vi "Configure Save File.vi"(0 "subVI":refnum<vi>, 2 "VI":refnum<vi>, 3 "ParentVI":refnum<vi>) -> (1 "Data Valid":bool)   [LabVIEW 2017]
doc: "Writes data to a LabVIEW measurement data file."
uses:
  <vilib>/express/express shared/ExFile.llb/ex_FileGlobals.vi
panel:
  in  "always hostless warning":string="The present target will not have a host connected.  When run, this VI will return an error."
  in  "maybe hostless warning":string="The present target may not always have a host connected.  When running hostless, this VI will return an error."
  in  "delimiter":string
  in  "x_columns":enum32{"none", "one", "multiple"}(radio)
  in  "overwrite_mode":T1(radio)
  in  "column headings":enum32{"one per segment", "once", "none"}(radio)
  in  "storage_format":enum32{"lvm", "tdm"}(radio)
  in  "delimiter enum":enum32{"tab", "comma"}(radio)
  in  "File path":path
  in  "Ask each iteration":bool
  in  "Ask only once":bool
  in  "Help":bool
  in  "Ok":bool
  in  "Cancel":bool
  in  "overwrite_mode_multi":i32
  in  "fixed_width":bool=TRUE
  in  "Width":i32=2 min=1 max=9
  in  "Samples":i32=1 min=1
  in  "Segments":i32=1 min=1
  in  "new_file_samples":bool
  in  "new_file_iter":bool
  in  "Time":i32 min=0 max=86399 format="%<%I:%M %p\n%m/%d/%y>T"
  in  "new_file_daily":bool
  in  "max_elapsed_seconds":i32 min=0 max=999
  in  "new_file_elaps_time":bool
  in  "KB":i32=100
  in  "new_file_size":bool=TRUE
  in  "Settings":bool
  in  "Save to series of files (multiple files)":bool
  in  "Save to one file":bool=TRUE
  in  "File Description":string
  in  "Ask user to choose file":bool
  in  "multi_file":bool
  in  "time_format_string":string="%Y-%m-%d"
  in  "new_file_mode":u16(ring)=2 items=["Date & Time", "Serial No.", "Both"]
  in  "File name":path=path "test.lvm"
  # "File Format"
  # "File Name"
  # "Action"
  # "Segment Headers"
  # "X Value Columns"
  # "If a file already exists"
  # "Delimiter"
  # "File Description"
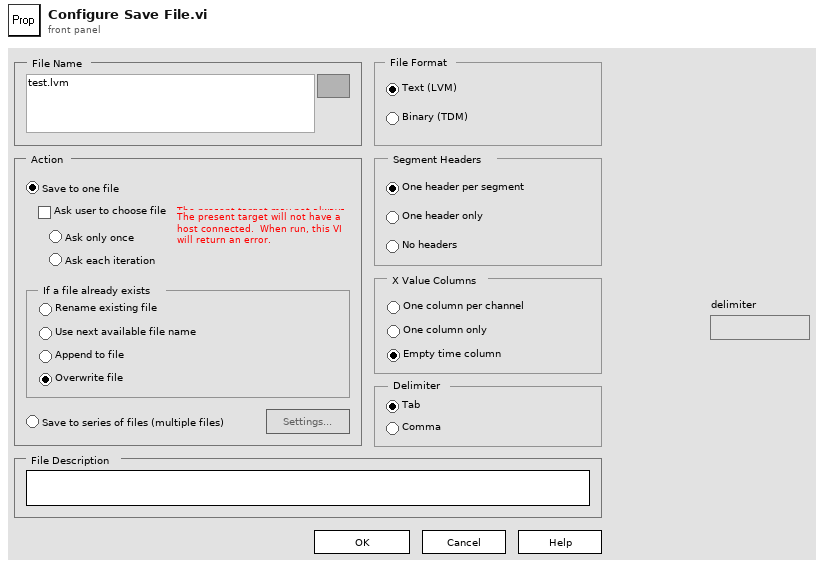
[diagram p1: front panel]
types:
  T1 = enum32{"overwrite", "overwrite & backup", "append", "next avail"}
  T2 = cluster{"Ctl Type":u16, "LV Express VI Ctl Label":string, "Wizard Ctl Label":string}[]
  T3 = typedef "propPageData.ctl" = cluster{"InstanceCtlRefs":refnum<vi>[], "ConfigDlgCtlRefs":refnum<vi>[], "Control Data":cluster{"Ctl Type":u16, "Instance Ctl Label":string, "Config Dialog Ctl Label":string}[], "viref Instance":refnum<vi>, "Types":i32[], "Config DialogVI":refnum<vi>}
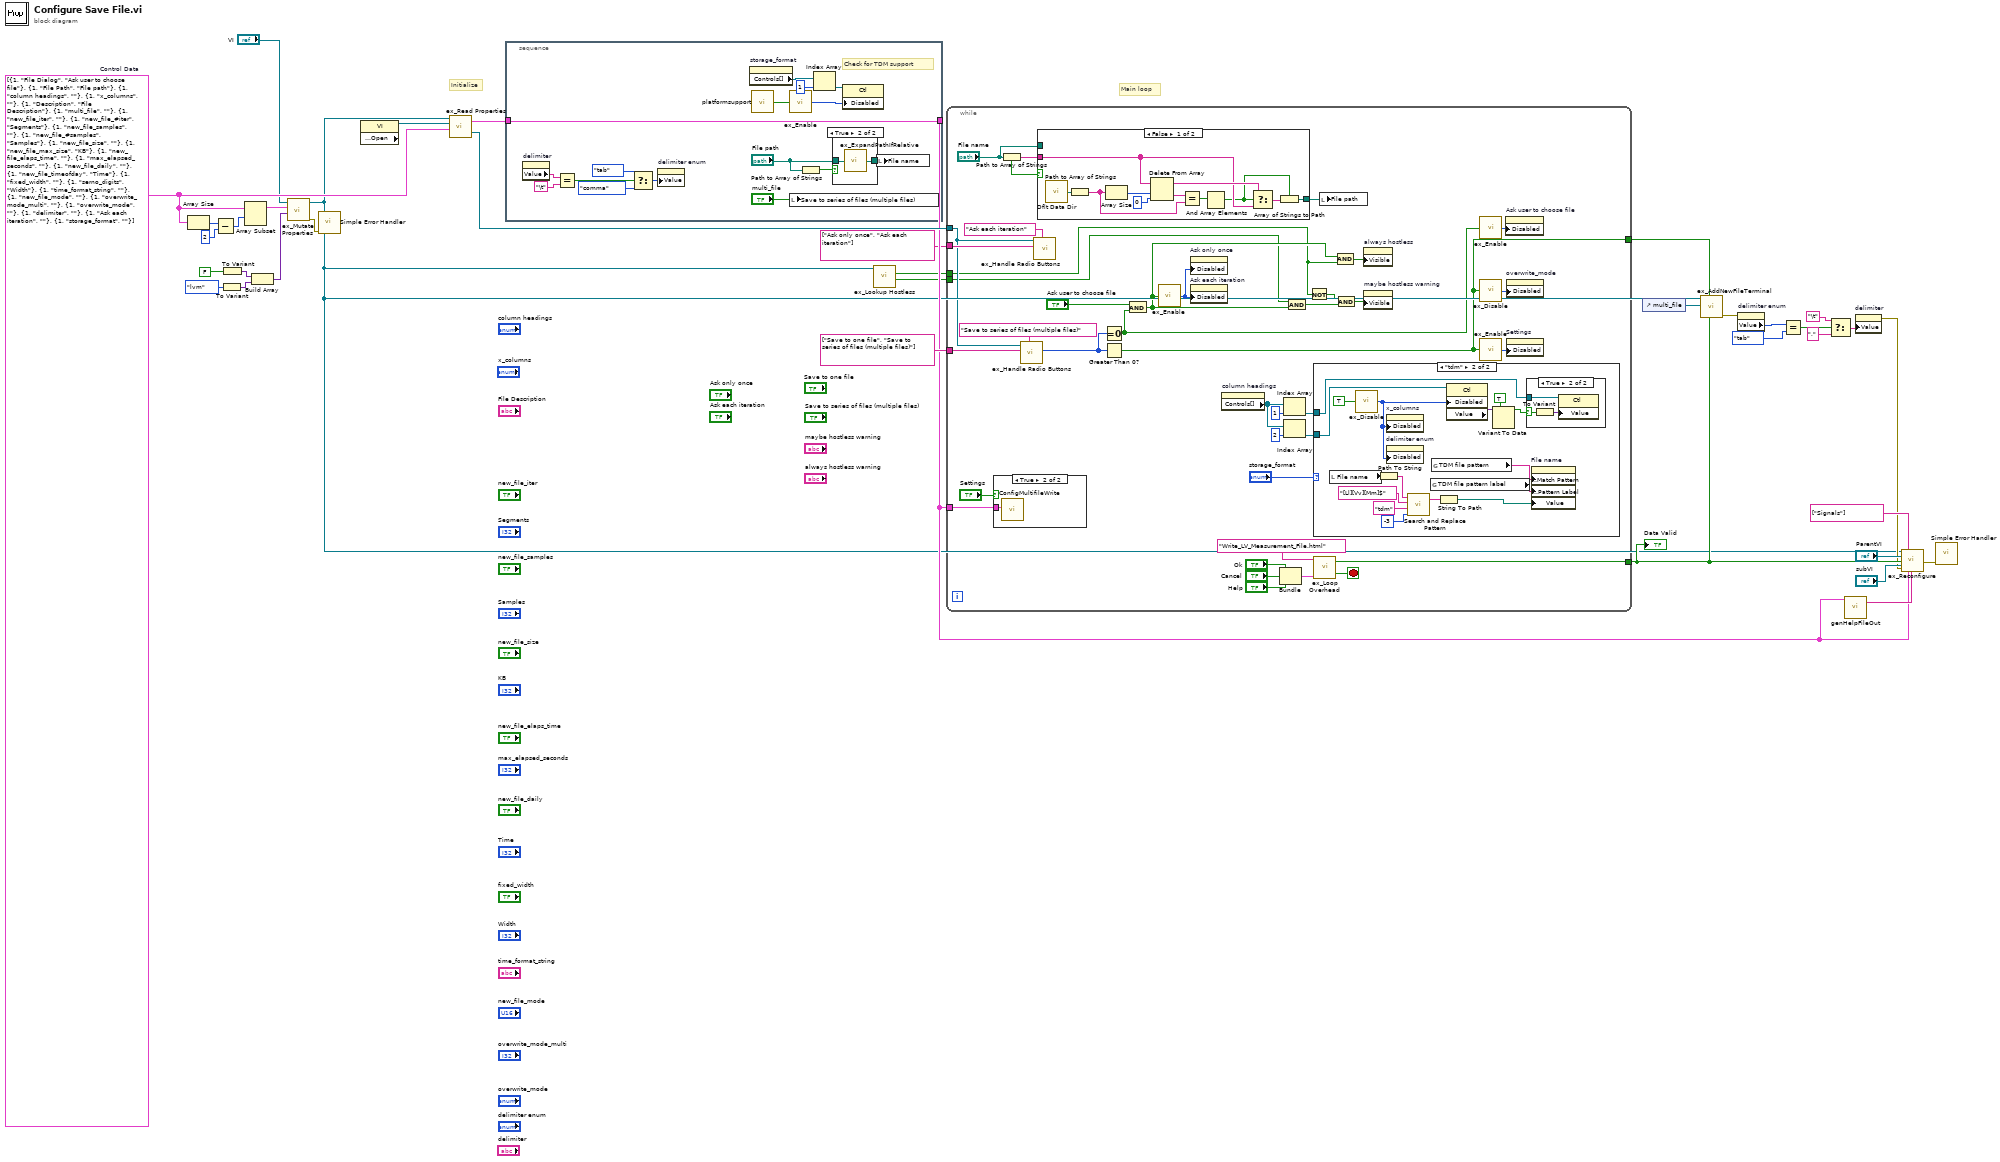
[diagram p0: block diagram]
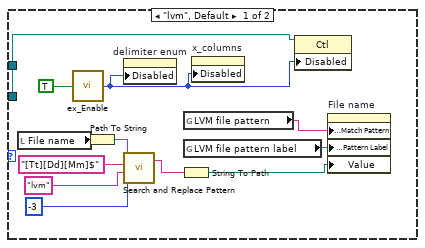
[diagram p3: hidden frame]
diagram:
  w13 = T2 [{"Ctl Type"=1, "LV Express VI Ctl Label"="File Dialog", "Wizard Ctl Label"="Ask user to choose file"}, {"Ctl Type"=1, "LV Express VI Ctl Label"="File Path", "Wizard Ctl Label"="File path"}, {"Ctl Type"=1, "LV Express VI Ctl Label"="column headings", "Wizard Ctl Label"=""}, {"Ctl Type"=1, "LV Express VI Ctl Label"="x_columns", "Wizard Ctl Label"=""}, {"Ctl Type"=1, "LV Express VI Ctl Label"="Description", "Wizard Ctl Label"="File Description"}, {"Ctl Type"=1, "LV Express VI Ctl Label"="multi_file", "Wizard Ctl Label"=""}, {"Ctl Type"=1, "LV Express VI Ctl Label"="new_file_iter", "Wizard Ctl Label"=""}, {"Ctl Type"=1, "LV Express VI Ctl Label"="new_file_#iter", "Wizard Ctl Label"="Segments"}, {"Ctl Type"=1, "LV Express VI Ctl Label"="new_file_samples", "Wizard Ctl Label"=""}, {"Ctl Type"=1, "LV Express VI Ctl Label"="new_file_#samples", "Wizard Ctl Label"="Samples"}, {"Ctl Type"=1, "LV Express VI Ctl Label"="new_file_size", "Wizard Ctl Label"=""}, {"Ctl Type"=1, "LV Express VI Ctl Label"="new_file_max_size", "Wizard Ctl Label"="KB"}, {"Ctl Type"=1, "LV Express VI Ctl Label"="new_file_elaps_time", "Wizard Ctl Label"=""}, {"Ctl Type"=1, "LV Express VI Ctl Label"="max_elapsed_seconds", "Wizard Ctl Label"=""}, {"Ctl Type"=1, "LV Express VI Ctl Label"="new_file_daily", "Wizard Ctl Label"=""}, {"Ctl Type"=1, "LV Express VI Ctl Label"="new_file_timeofday", "Wizard Ctl Label"="Time"}, {"Ctl Type"=1, "LV Express VI Ctl Label"="fixed_width", "Wizard Ctl Label"=""}, {"Ctl Type"=1, "LV Express VI Ctl Label"="serno_digits", "Wizard Ctl Label"="Width"}, {"Ctl Type"=1, "LV Express VI Ctl Label"="time_format_string", "Wizard Ctl Label"=""}, {"Ctl Type"=1, "LV Express VI Ctl Label"="new_file_mode", "Wizard Ctl Label"=""}, {"Ctl Type"=1, "LV Express VI Ctl Label"="overwrite_mode_multi", "Wizard Ctl Label"=""}, {"Ctl Type"=1, "LV Express VI Ctl Label"="overwrite_mode", "Wizard Ctl Label"=""}, {"Ctl Type"=1, "LV Express VI Ctl Label"="delimiter", "Wizard Ctl Label"=""}, {"Ctl Type"=1, "LV Express VI Ctl Label"="Ask each iteration", "Wizard Ctl Label"=""}, {"Ctl Type"=1, "LV Express VI Ctl Label"="storage_format", "Wizard Ctl Label"=""}]  # Control Data
  # "Initialize"
  # "Main loop"
  n1 = Array Size(array=w13) -> (size(s)=w12:i32)
  n2 = Subtract(x=w12, y=2) -> (x-y=w11:i32)
  n3 = To Variant(anything=enum32{"lvm", "tdm"}."lvm" ("storage_format")) -> (Variant=w5:variant)
  n4 = To Variant(anything=FALSE) -> (Variant=w1:variant)
  n5 = Array Subset(array=w13, index=w11) -> (w7:T2)  [unwired: 1 in]
  n6 = Build Array(w1, w5) -> (w4:variant[])
  n7 = call <vilib>:"ex_Mutate Properties.vi"("Control Values"=w4, "Control Data"=w7, "VI ref in"="VI") -> ("error out"=w3:errorcluster, "VI ref out"=w8:refnum<vi>)  [unwired: 7 out]
  n8 = call <vilib>:"Simple Error Handler.vi"("error in (no error)"=w3) -> ()  [unwired: 1 in, 8 out]
  n9 = property class="VI" props=["Front Panel Window:Open"]() -> (reference out=w24:refnum<vi>)  [unwired: 2 in, 2 out]
  n10 = call <vilib>:"ex_Read Properties.vi"("Control Data"=w13, "viref Configuration Dialog"=w24, "viref Instance"=w8) -> ("viref Configuration Dialog out"=w35:refnum<vi>, "Output Cluster"=w33:T3)  [unwired: 1 in, 2 out]
  n11 = stacked-sequence {
    tunnel: w33 -> [w53]
    tunnel: [w53] -> w28
    frame #0 {
      # "Check for TDM support"
      n12 = property on="delimiter" class="Str"() -> ("Value"=w43:string)  [unwired: 2 in, 2 out]
      n13 = Equal?(x=w43, y="\t") -> (x = y?=w40:bool)
      n14 = Select(t=enum32{"tab", "comma"}."tab" ("delimiter enum"), s=w40, f=enum32{"tab", "comma"}."comma" ("delimiter enum")) -> (s? t:f=w39:enum32{"tab", "comma"})
      n15 = property on="delimiter enum" class="RadioBtnsControl (strict)"("Value"=w39) -> ()  [unwired: 2 in, 2 out]
      n16 = property on="storage_format" class="RadioBtnsControl (strict)"() -> ("Controls[]"=w46:refnum<vi>[])  [unwired: 2 in, 2 out]
      n17 = call <vilib>:"platformsupport.vi"() -> ("TDM Support for Platform"=w48:bool)  [unwired: 1 out]
      n18 = call <vilib>:"ex_Enable.vi"("Enable?"=w48) -> ("Disabled Value"=w44:u8)
      n19 = local write "Save to series of files (multiple files)"("multi_file") -> ()
      n20 = Path to Array of Strings(0:"File path") -> (1:w50:bool)  [unwired: 1 out]
      n21 = Index Array(array=w46, index=1) -> (element=w45:refnum<vi>)
      n22 = case shown="True" w50 {
        tunnel: "File path" -> [w54 w56]
        tunnel: [w54 w55] -> w52
        frame False {
        }
        frame True {
          n23 = call <vilib>:"ex_ExpandPathIfRelative.vi"("Path"=w56) -> ("Expanded path"=w55:path)  [unwired: 4 out]
        }
      }
      n24 = property class="Ctl"(reference=w45, "Disabled"=w44) -> ()  [unwired: 1 in, 2 out]
      n25 = local write "File name"(w52) -> ()
    }
  }
  n26 = call <vilib>:"ex_Lookup Hostless.vi"("VI RefNum for Context"=w8) -> ("Maybe Hostless"=w14:bool, "Always Hostless"=w15:bool)  [unwired: 1 in, 8 out]
  n27 = while {
    tunnel: [w94] -> w31
    tunnel: w35 -> [w77]
    tunnel: string[] ["Save to one file", "Save to series of files (multiple files)"] ("Radio Buttons") -> [w95]
    tunnel: w28 -> [w93]
    tunnel: string[] ["Ask only once", "Ask each iteration"] ("Radio Buttons") -> [w83]
    tunnel: [w69] -> w26
    tunnel: w15 -> [w58]
    tunnel: w14 -> [w57]
    stop <- w92 stop-if-true
    n28 = case shown="True" "Settings" {
      tunnel: w93 -> [_ w139]
      frame False {
      }
      frame True {
        n29 = call <vilib>:"ConfigMultifileWrite.vi"("Reference"=w139) -> ()  [unwired: 11 out]
      }
    }
    n30 = Path to Array of Strings(0:"File name") -> (1:w80:bool, 2:w81:string[])
    n31 = call <vilib>:"ex_Handle Radio Buttons.vi"("Boolean Control"="Save to series of files (multiple files)" ("Numeric Control"), "Radio Buttons"=w95, "VI refnum"=w77) -> ("Selected Button"=w67:u32)  [unwired: 4 in, 4 out]
    n32 = call <vilib>:"ex_Handle Radio Buttons.vi"("Boolean Control"="Ask each iteration" ("Numeric Control"), "Radio Buttons"=w83, "VI refnum"=w77) -> ()  [unwired: 4 in, 5 out]
    n33 = case shown="False" w80 {
      tunnel: [w129 w138] -> w79
      tunnel: "File name" -> [_ w138]
      tunnel: w81 -> [w128 _]
      frame False {
        n34 = call <vilib>:"Dflt Data Dir.vi"() -> ("App:Default Data Directory"=w130:path)
        n35 = Path to Array of Strings(0:w130) -> (2:w137:string[])  [unwired: 1 out]
        n36 = Array Size(array=w137) -> (size(s)=w131:i32)
        n37 = Delete From Array(array=w128, length=w131, index=0) -> (deleted portion=w136:string[], array with subset deleted=w135:string[])
        n38 = Equal?(x=w136, y=w137) -> (x = y?=w133:bool[])
        n39 = And Array Elements(Boolean array=w133) -> (logical AND=w127:bool)
        n40 = Select(t=w135, s=w127, f=w128) -> (s? t:f=w134:string[])
        n41 = Array of Strings to Path(0:w134, 1:w127) -> (2:w129:path)
      }
      frame True {
      }
    }
    n42 = Equal To 0?(x=w67) -> (x = 0?=w65:bool)
    n43 = Greater Than 0?(x=w67) -> (x > 0?=w69:bool)
    n44 = And(x="Ask user to choose file", y=w65) -> (x .and. y?=w59:bool)
    n45 = call <vilib>:"ex_Enable.vi"("Enable?"=w59) -> ("Disabled Value"=w84:u8)
    n46 = property on="Ask only once" class="Bool (strict)"("Disabled"=w84) -> ()  [unwired: 2 in, 2 out]
    n47 = property on="Ask each iteration" class="Bool (strict)"("Disabled"=w84) -> ()  [unwired: 2 in, 2 out]
    n48 = property on="column headings" class="RadioBtnsControl (strict)"() -> ("Controls[]"=w72:refnum<vi>[])  [unwired: 2 in, 2 out]
    n49 = Bundle("Ok"="Ok", "Cancel"="Cancel", "Help"="Help") -> (w85:cluster{"Ok":bool, "Cancel":bool, "Help":bool})  [unwired: 1 out]
    n50 = Index Array(array=w72, index=1) -> (element=w70:refnum<vi>)
    n51 = Index Array(array=w72, index=2) -> (element=w73:refnum<vi>)
    n52 = And(x=w57, y=w59) -> (x .and. y?=w64:bool)
    n53 = Not(x=w58) -> (.not. x?=w63:bool)
    n54 = case shown="\"tdm\"" "storage_format" {
      tunnel: w73 -> [w107 w122]
      tunnel: w70 -> [_ w118]
      frame "lvm", Default {
        n55 = local read "File name"() -> (w105:path)
        n56 = call <vilib>:"ex_Enable.vi"("Enable?"=TRUE) -> ("Disabled Value"=w98:u8)
        n57 = Path To String(path=w105) -> (string=w104:string)
        n58 = property on="delimiter enum" class="RadioBtnsControl (strict)"("Disabled"=w98) -> ()  [unwired: 2 in, 2 out]
        n59 = call <vilib>:"Search and Replace Pattern.vi"("string"=w104, "regular expression (\"\")"="[Tt][Dd][Mm]$" ("regular expression (\"\")"), "replace string (\"\")"="lvm" ("replace string (\"\")"), "offset (0)"=-3) -> ("result string"=w100:string)  [unwired: 2 out]
        n60 = String To Path(string=w100) -> (path=w99:path)
        n61 = global read "ex_FileGlobals.vi" "LVM file pattern"() -> (w97:string)
        n62 = global read "ex_FileGlobals.vi" "LVM file pattern label"() -> (w96:string)
        n63 = property on="x_columns" class="RadioBtnsControl (strict)"("Disabled"=w98) -> ()  [unwired: 2 in, 2 out]
        n64 = property class="Ctl"(reference=w107, "Disabled"=w98) -> ()  [unwired: 1 in, 2 out]
        n65 = property on="File name" class="Path"("Browse Options:Match Pattern"=w97, "Browse Options:Pattern Label"=w96, "Value"=w99) -> ()  [unwired: 2 in, 2 out]
      }
      frame "tdm" {
        n66 = local read "File name"() -> (w117:path)
        n67 = call <vilib>:"ex_Disable.vi"("Disable?"=TRUE) -> ("Disabled value"=w110:u8)
        n68 = Path To String(path=w117) -> (string=w116:string)
        n69 = property on="x_columns" class="RadioBtnsControl (strict)"("Disabled"=w110) -> ()  [unwired: 2 in, 2 out]
        n70 = property on="delimiter enum" class="RadioBtnsControl (strict)"("Disabled"=w110) -> ()  [unwired: 2 in, 2 out]
        n71 = call <vilib>:"Search and Replace Pattern.vi"("string"=w116, "regular expression (\"\")"="[Ll][Vv][Mm]$" ("regular expression (\"\")"), "replace string (\"\")"="tdm" ("replace string (\"\")"), "offset (0)"=-3) -> ("result string"=w112:string)  [unwired: 2 out]
        n72 = global read "ex_FileGlobals.vi" "TDM file pattern label"() -> (w108:string)
        n73 = global read "ex_FileGlobals.vi" "TDM file pattern"() -> (w109:string)
        n74 = String To Path(string=w112) -> (path=w111:path)
        n75 = property class="Ctl"(reference=w122, "Disabled"=w110) -> ("Value"=w121:variant)  [unwired: 1 in, 2 out]
        n76 = Variant To Data(type=TRUE, Variant=w121) -> (data=w119:bool)  [unwired: 1 in, 1 out]
        n77 = case shown="True" w119 {
          selector: w119 -> [_ w125]
          tunnel: w118 -> [_ w126]
          frame False {
          }
          frame True {
            n78 = To Variant(anything=w125) -> (Variant=w124:variant)
            n79 = property class="Ctl"(reference=w126, "Value"=w124) -> ()  [unwired: 1 in, 2 out]
          }
        }
        n80 = property on="File name" class="Path"("Browse Options:Match Pattern"=w109, "Browse Options:Pattern Label"=w108, "Value"=w111) -> ()  [unwired: 2 in, 2 out]
      }
    }
    n81 = call <vilib>:"ex_Loop Overhead.vi"("Bottom Button Bar"=w85, "Help string to search for"="Write_LV_Measurement_File.html") -> ("Loop Terminator"=w92:bool, "Data Valid"=w94:bool)  [unwired: 1 in, 1 out]
    n82 = local write "File path"(w79) -> ()
    n83 = And(x=w59, y=w58) -> (x .and. y?=w61:bool)
    n84 = And(x=w63, y=w64) -> (x .and. y?=w62:bool)
    n85 = property on="always hostless" class="Str"("Visible"=w61) -> ()  [unwired: 2 in, 2 out]
    n86 = property on="maybe hostless warning" class="Str"("Visible"=w62) -> ()  [unwired: 2 in, 2 out]
    n87 = call <vilib>:"ex_Enable.vi"("Enable?"=w65) -> ("Disabled Value"=w66:u8)
    n88 = call <vilib>:"ex_Disable.vi"("Disable?"=w69) -> ("Disabled value"=w76:u8)
    n89 = call <vilib>:"ex_Enable.vi"("Enable?"=w69) -> ("Disabled Value"=w68:u8)
    n90 = property on="Ask user to choose file" class="Bool (strict)"("Disabled"=w66) -> ()  [unwired: 2 in, 2 out]
    n91 = property on="overwrite_mode" class="RadioBtnsControl (strict)"("Disabled"=w76) -> ()  [unwired: 2 in, 2 out]
    n92 = property on="Settings" class="Bool"("Disabled"=w68) -> ()  [unwired: 2 in, 2 out]
  }
  "Data Valid" <- w31
  n93 = control-ref of="multi_file"() -> (w25:refnum<vi>)
  n94 = call <vilib>:"ex_AddNewFileTerminal.vi"("Data Valid"=w31, "Boolean"=w26, "multi_file"=w25, "VI"=w8) -> ("error out"=w17:errorcluster)  [unwired: 1 in, 6 out]
  n95 = property on="delimiter enum" class="RadioBtnsControl (strict)"(error in=w17) -> ("Value"=w22:enum32{"tab", "comma"})  [unwired: 1 in, 2 out]
  n96 = Equal?(x=w22, y=enum32{"tab", "comma"}."tab" ("delimiter enum")) -> (x = y?=w23:bool)
  n97 = Select(t="\t", s=w23, f=",") -> (s? t:f=w18:string)
  n98 = call <vilib>:"genHelpFileOut.vi"("Output Cluster"=w28) -> ("Help Description"=w32:string)  [unwired: 5 out]
  n99 = property on="delimiter" class="Str"("Value"=w18) -> (error out=w16:errorcluster)  [unwired: 2 in, 1 out]
  n100 = call <vilib>:"ex_Reconfigure.vi"("VI refnum"=w8, "Parent VI refnum"="ParentVI", "Data Valid"=w31, "subVI refnum"="subVI", "error in"=w16, "Inputs/Outputs to Grow"=string[] ["Signals"] ("inputs"), "Props Cluster"=w28, "Configuration Description"=w32) -> ("error out"=w34:errorcluster)  [unwired: 5 in, 14 out]
  n101 = call <vilib>:"Simple Error Handler.vi"("error in (no error)"=w34) -> ()  [unwired: 1 in, 8 out]
